vi "rename VI.vi"(7 "Application":refnum<vi>, 8 "error in":errorcluster, 10 "new vi name":string, 11 "vi path":path) -> (0 "error out":errorcluster)   [LabVIEW 2013, in "scripting tools.lvlib"]
uses:
  scripting tools.lvlib
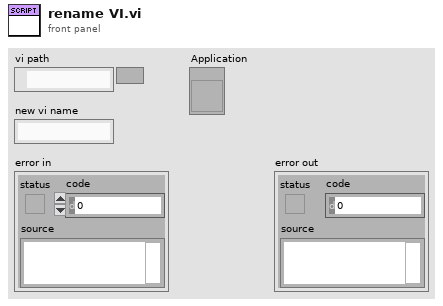
[diagram p1: front panel]
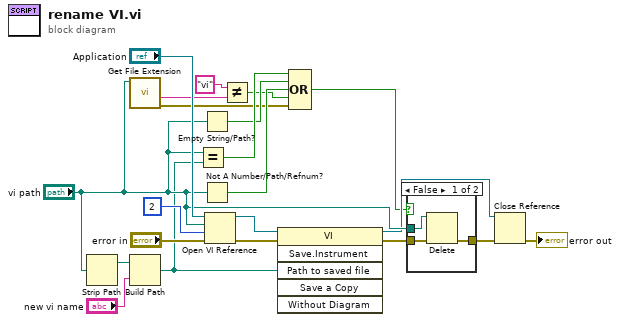
[diagram p0: block diagram]
diagram:
  n1 = Strip Path(path="vi path") -> (stripped path=w15:path)  [unwired: 1 out]
  n2 = call <vilib>:"Get File Extension.vi"("file"="vi path") -> ("error out"=w4:errorcluster, "filename without extension"=w3:string)  [unwired: 7 in, 2 out]
  n3 = Build Path(base path=w15, name or relative path="new vi name") -> (appended path=w8:path)
  n4 = Equal?(x="vi path", y=w8) -> (x = y?=w9:bool)
  n5 = Empty String/Path?(string/path="vi path") -> (empty?=w6:bool)
  n6 = Not A Number/Path/Refnum?(number/path/refnum="vi path") -> (NaN/Path/Refnum?=w5:bool)
  n7 = Open VI Reference(application reference (local)="Application", vi path="vi path", options=2 ("Template VIs as templates"), error in (no error)="error in") -> (vi reference=w16:refnum<vi>, error out=w13:errorcluster)  [unwired: 2 in]
  n8 = Not Equal?(x="vi", y=w3) -> (x != y?=w2:bool)
  n9 = invoke class="VI" method="Save.Instrument"(reference=w16, error in=w13, "Path to saved file"=w8) -> (reference out=w11:refnum<vi>, error out=w14:errorcluster)  [unwired: 3 in, 4 out]
  n10 = Compound Arithmetic op=OR(w9, w6, w5, w2, w4) -> (w7:bool)
  n11 = case shown="False" w7 {
    tunnel: "vi path" -> [w24 _]
    tunnel: w14 -> [w23 w25]
    tunnel: [w22 w25] -> w12
    frame False {
      n12 = Delete(path (use dialog)=w24, error in=w23) -> (error out=w22:errorcluster)  [unwired: 3 in, 2 out]
    }
    frame True {
    }
  }
  n13 = Close Reference(reference=w11, error in (no error)=w12) -> (error out=→"error out":errorcluster)
